vi "Run.vi"(8 "error in (no error)":errorcluster, 9 "s on last turn":dbl, 10 "Maze (0: Empty, -1: Enemy. >0: Teammate":i32[][](array[numeric]), 11 "Scout In":refnum<class "Protector.lvclass">) -> (0 "error out":errorcluster, 1 "Direction":T1, 2 "Action":T2, 3 "Scout Out":refnum<class "Protector.lvclass">, 4 "Replicated":refnum<class "Square.lvclass">)   [LabVIEW 2015, in "Protector.lvclass"]
uses:
  Protector.lvclass
  Type Defs/Action Enum.ctl
  Type Defs/Direction Enum.ctl
  Square/Square.lvclass
  Formics/Attack Options.ctl
  Formics/Formics.lvclass/Formics.ctl
  Formics/Formics.lvclass
panel:
  out "Map":i32[](array[numeric])
  in  "Status":string
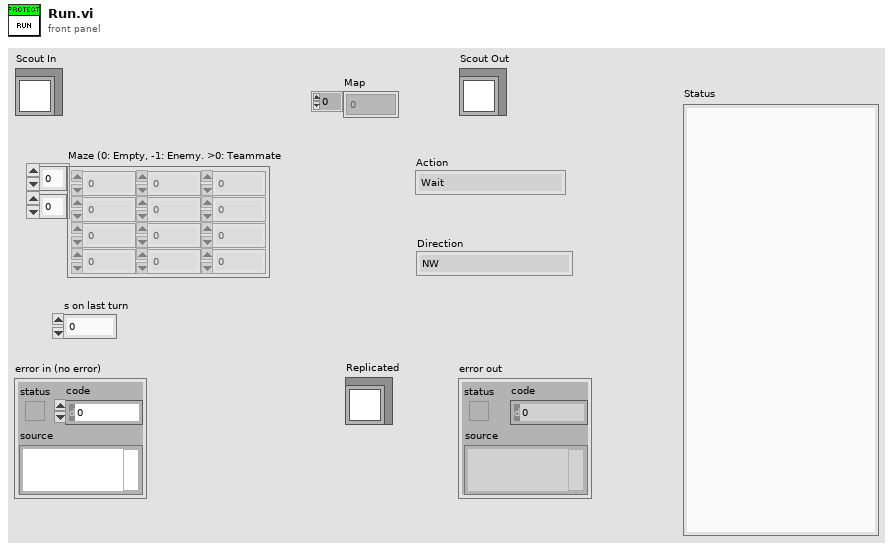
[diagram p1: front panel]
types:
  T1 = typedef "Square.lvclass/Direction Enum.ctl" = enum16{"NW", "N", "NE", "E", "SE", "S", "SW", "W"}
  T2 = typedef "Square.lvclass/Action Enum.ctl" = enum16{"Wait", "Move", "Attack", "Replicate"}
  T3 = typedef "Formics.lvclass/Attack Options.ctl" = enum16{"Attack", "Run", "Distract"}
  T4 = typedef "Formics.lvclass/Kamikaze DVR.ctl" = refnum<data-value>
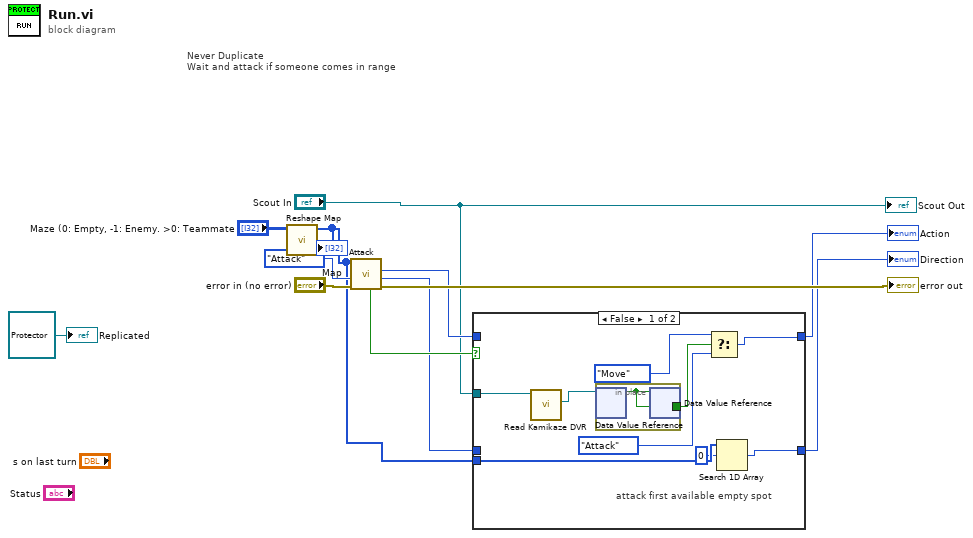
[diagram p0: block diagram]
diagram:
  # "Never Duplicate\nWait and attack if someone comes in range"
  n1 = call "Reshape Map.vi"("Maze (0: Empty, -1: Enemy. >0: Teammate"="Maze (0: Empty, -1: Enemy. >0: Teammate") -> ("Map"=w1:i32[])  [unwired: 9 in, 1 out]
  "Map" <- w1
  n2 = call "Attack.vi"("error in (no error)"="error in (no error)", "Attack?"=Attack_Options."Attack", "Maze (0: Empty, -1: Enemy. >0: Teammate"=w1) -> ("error out"=→"error out":errorcluster, "Direction"=w4:i32, "Action"=w6:T2, "Enemy Found?"=w7:bool)  [unwired: 3 in, 2 out]
  n3 = case shown="False" w7 {
    tunnel: w6 -> [_ w24]
    tunnel: w4 -> [_ w23]
    tunnel: [w18 w24] -> w5
    tunnel: [w14 w23] -> w3
    tunnel: "Scout In" -> [w21 _]
    tunnel: w1 -> [w15 _]
    frame False {
      # "attack first available empty spot"
      n4 = call "Read Kamikaze DVR.vi"("Mother in"=w21) -> ("Kamikaze DVR"=w20:T4)  [unwired: 8 in, 2 out]
      n5 = in-place {
        in-place-border: [w22] -> w17
        n6 = in-place-dvr #1(w20) -> (w22:bool)  [unwired: 1 out]
        n7 = in-place-dvr #1(w22) -> ()  [unwired: 2 out]
      }
      n8 = Select(t=Action_Enum."Move" ("Action"), s=w17, f=Action_Enum."Attack" ("t")) -> (s? t:f=w18:T2)
      n9 = Search 1D Array(1D array=w15, element=0) -> (index of element=w14:i32)  [unwired: 1 in]
    }
    frame True {
    }
  }
  "Action" <- w5
  "Direction" <- w3
  "Scout Out" <- "Scout In"
  "Replicated" <- refnum<class "Protector.lvclass"> refnum ("Replicated")
